vi "test_read-nmea-data2.vi"() -> ()   [LabVIEW 2019] (continued)
11,72,359,,2*70\n\t\n15:13:45.63\tF9P\t$GAGSV,2,2,08,12,40,103,,19,26,045,,25,09,249,,36,26,308,,2*7D\n\t\n15:13:45.65\tF9P\t$GBGSV,1,1,04,11,49,132,32,14,87,114,28,28,,,30,33,61,220,27,1*41\n\t\n15:13:45.67\tF9P\t$GBGSV,1,1,03,11,49,132,,14,87,114,27,33,61,220,,3*46\n\t\n15:13:45.69\tF9P\t$GNGLL,3723.57229,N,12656.98820,E,061347.00,A,A*73\n\t\n15:13:45.71\tF9P\t\t\n15:13:45.73\tF9P\t\t\n15:13:45.75\tF9P\t\t\n15:13:45.77\tF9P\t\t\n15:13:45.79\tF9P\t\t\n15:13:45.81\tF9P\t\t\n15:13:45.83\tF9P\t\t\n15:13:45.85\tF9P\t\t\n15:13:45.87\tF9P\t\t\n15:13:45.89\tF9P\t\t\n15:13:45.91\tF9P\t\t\n15:13:45.93\tF9P\t\t\n15:13:45.95\tF9P\t\t\n15:13:45.97\tF9P\t\t\n15:13:45.99\tF9P\t\t\n15:13:46.01\tF9P\t\t\n15:13:46.03\tF9P\t\t\n15:13:46.05\tF9P\t\t\n15:13:46.07\tF9P\t\t\n15:13:46.09\tF9P\t\t\n15:13:46.11\tF9P\t\t\n15:13:46.13\tF9P\t\t\n15:13:46.15\tF9P\t\t\n15:13:46.17\tF9P\t\t\n15:13:46.19\tF9P\t\t\n15:13:46.21\tF9P\t\t\n15:13:46.23\tF9P\t$GNRMC,061348.00,A,3723.57290,N,12656.98771,E,2.680,332.74,250720,,,A,V*07\n\t\n15:13:46.25\tF9P\t$GNVTG,332.74,T,,M,2.680,N,4.963,K,A*26\n\t\n15:13:46.27\tF9P\t$GNGGA,061348.00,3723.57290,N,12656.98771,E,1,12,0.78,48.0,M,18.5,M,,*7C\n\t\n15:13:46.29\tF9P\t$GNGSA,A,3,12,06,19,05,17,09,04,02,,,,,1.48,0.78,1.25,1*04\n\t\n15:13:46.31\tF9P\t$GNGSA,A,3,85,70,71,84,,,,,,,,,1.48,0.78,1.25,2*06\n\t\n15:13:46.33\tF9P\t$GNGSA,A,3,36,19,11,04,09,12,,,,,,,1.48,0.78,1.25,3*04\n\t\n15:13:46.35\tF9P\t$GNGSA,A,3,14,11,33,,,,,,,,,,1.48,0.78,1.25,4*05\n\t\n15:13:46.37\tF9P\t$GPGSV,3,1,09,02,55,320,32,04,17,043,25,05,38,248,28,06,64,050,31,1*66\n\t\n15:13:46.39\tF9P\t$GPGSV,3,2,09,09,44,073,30,12,23,276,41,17,32,154,36,19,51,157,34,1*6C\n\t\n15:13:46.41\tF9P\t$GPGSV,3,3,09,25,12,306,19,1*54\n\t\n15:13:46.43\tF9P\t$GPGSV,3,1,09,02,55,320,,04,17,043,14,05,38,248,18,06,64,050,24,6*65\n\t\n15:13:46.45\tF9P\t$GPGSV,3,2,09,09,44,073,24,12,23,276,22,17,32,154,22,19,51,157,,6*69\n\t\n15:13:46.47\tF9P\t$GPGSV,3,3,09,25,12,306,,6*5B\n\t\n15:13:46.49\tF9P\t$GLGSV,2,1,08,69,11,031,36,70,70,038,25,71,53,206,26,72,05,210,18,1*7D\n\t\n15:13:46.51\tF9P\t$GLGSV,2,2,08,77,01,325,,84,19,123,23,85,70,070,32,86,37,330,,1*76\n\t\n15:13:46.53\tF9P\t$GLGSV,2,1,08,69,11,031,25,70,70,038,,71,53,206,16,72,05,210,,3*70\n\t\n15:13:46.55\tF9P\t$GLGSV,2,2,08,77,01,325,,84,19,123,30,85,70,070,22,86,37,330,,3*77\n\t\n15:13:46.57\tF9P\t$GAGSV,2,1,08,02,08,297,10,04,66,116,32,09,32,193,24,11,72,359,26,7*77\n\t\n15:13:46.59\tF9P\t$GAGSV,2,2,08,12,40,103,25,19,26,045,16,25,09,249,19,36,26,308,17,7*76\n\t\n15:13:46.61\tF9P\t$GAGSV,2,1,08,02,08,297,,04,66,116,,09,32,193,,11,72,359,,2*70\n\t\n15:13:46.63\tF9P\t$GAGSV,2,2,08,12,40,103,,19,26,045,,25,09,249,,36,26,308,,2*7D\n\t\n15:13:46.65\tF9P\t$GBGSV,1,1,04,11,49,132,32,14,87,114,28,28,,,30,33,61,220,29,1*4F\n\t\n15:13:46.67\tF9P\t$GBGSV,1,1,03,11,49,132,31,14,87,114,27,33,61,220,,3*44\n\t\n15:13:46.69\tF9P\t$GNGLL,3723.57290,N,12656.98771,E,061348.00,A,A*75\n\t\n15:13:46.71\tF9P\t\t\n15:13:46.73\tF9P\t\t\n15:13:46.75\tF9P\t\t\n15:13:46.77\tF9P\t\t\n15:13:46.79\tF9P\t\t\n15:13:46.81\tF9P\t\t\n15:13:46.83\tF9P\t\t\n15:13:46.85\tF9P\t\t\n15:13:46.87\tF9P\t\t\n15:13:46.89\tF9P\t\t\n15:13:46.91\tF9P\t\t\n15:13:46.93\tF9P\t\t\n15:13:46.95\tF9P\t\t\n15:13:46.97\tF9P\t\t\n15:13:46.99\tF9P\t\t\n15:13:47.01\tF9P\t\t\n15:13:47.03\tF9P\t\t\n15:13:47.05\tF9P\t\t\n15:13:47.07\tF9P\t\t\n15:13:47.09\tF9P\t\t\n15:13:47.11\tF9P\t\t\n15:13:47.13\tF9P\t\t\n15:13:47.15\tF9P\t\t\n15:13:47.17\tF9P\t\t\n15:13:47.19\tF9P\t\t\n15:13:47.21\tF9P\t\t\n15:13:47.23\tF9P\t$GNRMC,061349.00,A,3723.57353,N,12656.98784,E,2.463,343.29,250720,,,A,V*03\n\t\n15:13:47.25\tF9P\t$GNVTG,343.29,T,,M,2.463,N,4.562,K,A*2A\n\t\n15:13:47.27\tF9P\t$GNGGA,061349.00,3723.57353,N,12656.98784,E,1,12,0.67,48.9,M,18.5,M,,*7E\n\t\n15:13:47.29\tF9P\t$GNGSA,A,3,12,06,19,05,17,09,04,02,,,,,1.24,0.67,1.04,1*03\n\t\n15:13:47.31\tF9P\t$GNGSA,A,3,85,70,71,84,,,,,,,,,1.24,0.67,1.04,2*01\n\t\n15:13:47.33\tF9P\t$GNGSA,A,3,36,19,11,04,09,12,,,,,,,1.24,0.67,1.04,3*03\n\t\n15:13:47.35\tF9P\t$GNGSA,A,3,14,11,33,,,,,,,,,,1.24,0.67,1.04,4*02\n\t\n15:13:47.37\tF9P\t$GPGSV,3,1,09,02,55,320,29,04,17,043,25,05,38,248,29,06,64,050,32,1*6E\n\t\n15:13:47.39\tF9P\t$GPGSV,3,2,09,09,44,073,25,12,23,276,41,17,32,154,28,19,51,157,37,1*64\n\t\n15:13:47.41\tF9P\t$GPGSV,3,3,09,25,12,306,18,1*55\n\t\n15:13:47.43\tF9P\t$GPGSV,3,1,09,02,55,320,,04,17,043,,05,38,248,18,06,64,050,25,6*61\n\t\n15:13:47.45\tF9P\t$GPGSV,3,2,09,09,44,073,25,12,23,276,24,17,32,154,22,19,51,157,,6*6E\n\t\n15:13:47.47\tF9P\t$GPGSV,3,3,09,25,12,306,,6*5B\n\t\n15:13:47.49\tF9P\t$GLGSV,2,1,08,69,11,031,31,70,70,038,24,71,53,206,26,72,05,210,19,1*7A\n\t\n15:13:47.51\tF9P\t$GLGSV,2,2,08,77,01,325,,84,19,123,24,85,70,070,31,86,37,330,,1*72\n\t\n15:13:47.53\tF9P\t$GLGSV,2,1,08,69,11,031,22,70,70,038,,71,53,206,15,72,05,210,,3*74\n\t\n15:13:47.55\tF9P\t$GLGSV,2,2,08,77,01,325,,84,19,123,22,85,70,070,22,86,37,330,,3*74\n\t\n15:13:47.57\tF9P\t$GAGSV,2,1,08,02,08,297,06,04,66,116,37,09,32,193,23,11,72,359,25,7*71\n\t\n15:13:47.59\tF9P\t$GAGSV,2,2,08,12,40,103,32,19,26,045,17,25,09,249,15,36,26,308,13,7*79\n\t\n15:13:47.61\tF9P\t$GAGSV,2,1,08,02,08,297,,04,66,116,,09,32,193,,11,72,359,,2*70\n\t\n15:13:47.63\tF9P\t$GAGSV,2,2,08,12,40,103,,19,26,045,,25,09,249,,36,26,308,,2*7D\n\t\n15:13:47.65\tF9P\t$GBGSV,1,1,04,11,49,132,27,14,87,114,28,28,,,30,33,61,220,38,1*4B\n\t\n15:13:47.67\tF9P\t$GBGSV,1,1,03,11,49,132,27,14,87,114,,33,61,220,,3*46\n\t\n15:13:47.69\tF9P\t$GNGLL,3723.57353,N,12656.98784,E,061349.00,A,A*70\n\t\n15:13:47.71\tF9P\t\t\n15:13:47.73\tF9P\t\t\n15:13:47.75\tF9P\t\t\n15:13:47.77\tF9P\t\t\n15:13:47.79\tF9P\t\t\n15:13:47.81\tF9P\t\t\n15:13:47.83\tF9P\t\t\n15:13:47.85\tF9P\t\t\n15:13:47.87\tF9P\t\t\n15:13:47.89\tF9P\t\t\n15:13:47.91\tF9P\t\t\n15:13:47.93\tF9P\t\t\n15:13:47.95\tF9P\t\t\n15:13:47.97\tF9P\t\t\n15:13:47.99\tF9P\t\t\n15:13:48.01\tF9P\t\t\n15:13:48.03\tF9P\t\t\n15:13:48.05\tF9P\t\t\n15:13:48.07\tF9P\t\t\n15:13:48.09\tF9P\t\t\n15:13:48.11\tF9P\t\t\n15:13:48.13\tF9P\t\t\n15:13:48.15\tF9P\t\t\n15:13:48.17\tF9P\t\t\n15:13:48.19\tF9P\t\t\n15:13:48.21\tF9P\t\t\n15:13:48.23\tF9P\t$GNRMC,061350.00,A,3723.57391,N,12656.98799,E,1.815,345.24,250720,,,A,V*0C\n\t\n15:13:48.25\tF9P\t$GNVTG,345.24,T,,M,1.815,N,3.361,K,A*2D\n\t\n15:13:48.27\tF9P\t$GNGGA,061350.00,3723.57391,N,12656.98799,E,1,12,0.75,49.6,M,18.5,M,,*79\n\t\n15:13:48.29\tF9P\t$GNGSA,A,3,12,06,19,05,17,09,04,02,,,,,1.37,0.75,1.15,1*02\n\t\n15:13:48.31\tF9P\t$GNGSA,A,3,85,70,71,84,,,,,,,,,1.37,0.75,1.15,2*00\n\t\n15:13:48.33\tF9P\t$GNGSA,A,3,36,19,11,04,09,12,,,,,,,1.37,0.75,1.15,3*02\n\t\n15:13:48.35\tF9P\t$GNGSA,A,3,14,11,33,,,,,,,,,,1.37,0.75,1.15,4*03\n\t\n15:13:48.37\tF9P\t$GPGSV,3,1,09,02,55,320,30,04,17,043,25,05,38,248,24,06,64,050,27,1*6F\n\t\n15:13:48.39\tF9P\t$GPGSV,3,2,09,09,44,073,32,12,23,276,34,17,32,154,36,19,51,157,32,1*6A\n\t\n15:13:48.41\tF9P\t$GPGSV,3,3,09,25,12,306,18,1*55\n\t\n15:13:48.43\tF9P\t$GPGSV,3,1,09,02,55,320,,04,17,043,,05,38,248,17,06,64,050,24,6*6F\n\t\n15:13:48.45\tF9P\t$GPGSV,3,2,09,09,44,073,25,12,23,276,24,17,32,154,21,19,51,157,,6*6D\n\t\n15:13:48.47\tF9P\t$GPGSV,3,3,09,25,12,306,,6*5B\n\t\n15:13:48.49\tF9P\t$GLGSV,2,1,08,69,11,031,29,70,70,038,25,71,53,206,27,72,05,210,19,1*73\n\t\n15:13:48.51\tF9P\t$GLGSV,2,2,08,77,01,325,,84,19,123,25,85,70,070,31,86,37,330,,1*73\n\t\n15:13:48.53\tF9P\t$GLGSV,2,1,08,69,11,031,21,70,70,038,,71,53,206,14,72,05,210,,3*76\n\t\n15:13:48.55\tF9P\t$GLGSV,2,2,08,77,01,325,,84,19,123,23,85,70,070,21,86,37,330,,3*76\n\t\n15:13:48.57\tF9P\t$GAGSV,2,1,08,02,08,297,10,04,66,116,36,09,32,193,22,11,72,359,25,7*76\n\t\n15:13:48.59\tF9P\t$GAGSV,2,2,08,12,40,103,30,19,26,045,16,25,09,249,14,36,26,308,12,7*7A\n\t\n15:13:48.61\tF9P\t$GAGSV,2,1,08,02,08,297,,04,66,116,,09,32,193,,11,72,359,,2*70\n\t\n15:13:48.63\tF9P\t$GAGSV,2,2,08,12,40,103,,19,26,045,,25,09,249,,36,26,308,,2*7D\n\t\n15:13:48.65\tF9P\t$GBGSV,1,1,04,11,49,132,32,14,87,114,28,28,,,35,33,61,220,33,1*41\n\t\n15:13:48.67\tF9P\t$GBGSV,1,1,03,11,49,132,26,14,87,114,,33,61,220,,3*47\n\t\n15:13:48.69\tF9P\t$GNGLL,3723.57391,N,12656.98799,E,061350.00,A,A*7A\n\t\n15:13:48.71\tF9P\t\t\n15:13:48.73\tF9P\t\t\n15:13:48.75\tF9P\t\t\n15:13:48.77\tF9P\t\t\n15:13:48.79\tF9P\t\t\n15:13:48.81\tF9P\t\t\n15:13:48.83\tF9P\t\t\n15:13:48.85\tF9P\t\t\n15:13:48.87\tF9P\t\t\n15:13:48.89\tF9P\t\t\n15:13:48.91\tF9P\t\t\n15:13:48.93\tF9P\t\t\n15:13:48.95\tF9P\t\t\n15:13:48.97\tF9P\t\t\n15:13:48.99\tF9P\t\t\n15:13:49.01\tF9P\t\t\n15:13:49.03\tF9P\t\t\n15:13:49.05\tF9P\t\t\n15:13:49.07\tF9P\t\t\n15:13:49.09\tF9P\t\t\n15:13:49.11\tF9P\t\t\n15:13:49.13\tF9P\t\t\n15:13:49.15\tF9P\t\t\n15:13:49.17\tF9P\t\t\n15:13:49.19\tF9P\t\t\n15:13:49.21\tF9P\t\t\n15:13:49.23\tF9P\t$GNRMC,061351.00,A,3723.57445,N,12656.98793,E,1.823,343.63,250720,,,A,V*09\n\t\n15:13:49.25\tF9P\t$GNVTG,343.63,T,,M,1.823,N,3.376,K,A*2B\n\t\n15:13:49.27\tF9P\t$GNGGA,061351.00,3723.57445,N,12656.98793,E,1,12,0.70,49.5,M,18.5,M,,*7A\n\t\n15:13:49.29\tF9P\t$GNGSA,A,3,12,06,19,05,17,09,04,02,,,,,1.27,0.70,1.06,1*04\n\t\n15:13:49.31\tF9P\t$GNGSA,A,3,85,70,71,84,,,,,,,,,1.27,0.70,1.06,2*06\n\t\n15:13:49.33\tF9P\t$GNGSA,A,3,36,19,11,04,09,12,,,,,,,1.27,0.70,1.06,3*04\n\t\n15:13:49.35\tF9P\t$GNGSA,A,3,14,11,33,,,,,,,,,,1.27,0.70,1.06,4*05\n\t\n15:13:49.37\tF9P\t$GPGSV,3,1,09,02,55,320,29,04,17,043,25,05,38,248,34,06,64,050,28,1*69\n\t\n15:13:49.39\tF9P\t$GPGSV,3,2,09,09,44,073,28,12,23,276,33,17,32,154,29,19,51,157,36,1*6C\n\t\n15:13:49.41\tF9P\t$GPGSV,3,3,09,25,12,306,21,1*5F\n\t\n15:13:49.43\tF9P\t$GPGSV,3,1,09,02,55,320,,04,17,043,,05,38,248,17,06,64,050,22,6*69\n\t\n15:13:49.45\tF9P\t$GPGSV,3,2,09,09,44,073,24,12,23,276,22,17,32,154,20,19,51,157,,6*6B\n\t\n15:13:49.47\tF9P\t$GPGSV,3,3,09,25,12,306,,6*5B\n\t\n15:13:49.49\tF9P\t$GLGSV,2,1,08,69,11,031,30,70,70,038,24,71,53,206,27,72,05,210,18,1*7B\n\t\n15:13:49.51\tF9P\t$GLGSV,2,2,08,77,01,325,,84,19,123,24,85,70,070,27,86,37,330,,1*75\n\t\n15:13:49.53\tF9P\t$GLGSV,2,1,08,69,11,031,21,70,70,038,,71,53,206,14,72,05,210,,3*76\n\t\n15:13:49.55\tF9P\t$GLGSV,2,2,08,77,01,325,,84,19,123,24,85,70,070,21,86,37,330,,3*71\n\t\n15:13:49.57\tF9P\t$GAGSV,2,1,08,02,08,296,09,04,66,116,30,09,32,193,22,11,72,359,24,7*78\n\t\n15:13:49.59\tF9P\t$GAGSV,2,2,08,12,40,103,34,19,26,045,16,25,09,249,13,36,26,308,12,7*79\n\t\n15:13:49.61\tF9P\t$GAGSV,2,1,08,02,08,296,,04,66,116,,09,32,193,,11,72,359,,2*71\n\t\n15:13:49.63\tF9P\t$GAGSV,2,2,08,12,40,103,,19,26,045,,25,09,249,,36,26,308,,2*7D\n\t\n15:13:49.65\tF9P\t$GBGSV,1,1,04,11,49,132,39,14,87,114,28,28,,,27,33,61,220,39,1*43\n\t\n15:13:49.67\tF9P\t$GBGSV,1,1,03,11,49,132,,14,87,114,,33,61,220,,3*43\n\t\n15:13:49.69\tF9P\t$GNGLL,3723.57445,N,12656.98793,E,061351.00,A,A*7F\n\t\n15:13:49.71\tF9P\t\t\n15:13:49.73\tF9P\t\t\n15:13:49.75\tF9P\t\t\n15:13:49.77\tF9P\t\t\n15:13:49.79\tF9P\t\t\n15:13:49.81\tF9P\t\t\n15:13:49.83\tF9P\t\t\n15:13:49.85\tF9P\t\t\n15:13:49.87\tF9P\t\t\n15:13:49.89\tF9P\t\t\n15:13:49.91\tF9P\t\t\n15:13:49.93\tF9P\t\t\n15:13:49.95\tF9P\t\t\n15:13:49.97\tF9P\t\t\n15:13:49.99\tF9P\t\t\n15:13:50.01\tF9P\t\t\n15:13:50.03\tF9P\t\t\n15:13:50.05\tF9P\t\t\n15:13:50.07\tF9P\t\t\n15:13:50.09\tF9P\t\t\n15:13:50.11\tF9P\t\t\n15:13:50.13\tF9P\t\t\n15:13:50.15\tF9P\t\t\n15:13:50.17\tF9P\t\t\n15:13:50.19\tF9P\t\t\n15:13:50.21\tF9P\t\t\n15:13:50.23\tF9P\t$GNRMC,061352.00,A,3723.57495,N,12656.98774,E,1.787,343.52,250720,,,A,V*0D\n\t\n15:13:50.25\tF9P\t$GNVTG,343.52,T,,M,1.787,N,3.310,K,A*28\n\t\n15:13:50.27\tF9P\t$GNGGA,061352.00,3723.57495,N,12656.98774,E,1,12,0.81,49.2,M,18.5,M,,*74\n\t\n15:13:50.29\tF9P\t$GNGSA,A,3,12,06,19,05,17,09,04,02,,,,,1.45,0.81,1.20,1*0A\n\t\n15:13:50.31\tF9P\t$GNGSA,A,3,85,70,71,84,,,,,,,,,1.45,0.81,1.20,2*08\n\t\n15:13:50.33\tF9P\t$GNGSA,A,3,36,19,11,04,09,12,,,,,,,1.45,0.81,1.20,3*0A\n\t\n15:13:50.35\tF9P\t$GNGSA,A,3,14,11,33,,,,,,,,,,1.45,0.81,1.20,4*0B\n\t\n15:13:50.37\tF9P\t$GPGSV,3,1,09,02,55,320,30,04,17,043,24,05,38,248,,06,64,050,29,1*66\n\t\n15:13:50.39\tF9P\t$GPGSV,3,2,09,09,44,073,29,12,23,276,32,17,32,154,33,19,51,157,41,1*67\n\t\n15:13:50.41\tF9P\t$GPGSV,3,3,09,25,12,306,24,1*5A\n\t\n15:13:50.43\tF9P\t$GPGSV,3,1,09,02,55,320,,04,17,043,,05,38,248,15,06,64,050,23,6*6A\n\t\n15:13:50.45\tF9P\t$GPGSV,3,2,09,09,44,073,22,12,23,276,21,17,32,154,19,19,51,157,,6*64\n\t\n15:13:50.47\tF9P\t$GPGSV,3,3,09,25,12,306,,6*5B\n\t\n15:13:50.49\tF9P\t$GLGSV,2,1,08,69,11,031,31,70,70,038,24,71,53,206,32,72,05,210,18,1*7E\n\t\n15:13:50.51\tF9P\t$GLGSV,2,2,08,77,01,325,,84,19,123,25,85,70,070,32,86,37,330,,1*70\n\t\n15:13:50.53\tF9P\t$GLGSV,2,1,08,69,11,031,23,70,70,038,,71,53,206,16,72,05,210,,3*76\n\t\n15:13:50.55\tF9P\t$GLGSV,2,2,08,77,01,325,,84,19,123,26,85,70,070,19,86,37,330,,3*78\n\t\n15:13:50.57\tF9P\t$GAGSV,2,1,08,02,08,296,09,04,66,116,28,09,32,193,20,11,72,359,26,7*71\n\t\n15:13:50.59\tF9P\t$GAGSV,2,2,08,12,40,103,29,19,26,045,15,25,09,249,13,36,26,308,10,7*74\n\t\n15:13:50.61\tF9P\t$GAGSV,2,1,08,02,08,296,,04,66,116,,09,32,193,,11,72,359,,2*71\n\t\n15:13:50.63\tF9P\t$GAGSV,2,2,08,12,40,103,,19,26,045,,25,09,249,,36,26,308,,2*7D\n\t\n15:13:50.65\tF9P\t$GBGSV,1,1,04,11,49,132,37,14,87,114,29,28,,,32,33,61,220,29,1*49\n\t\n15:13:50.67\tF9P\t$GBGSV,1,1,03,11,49,132,29,14,87,114,,33,61,220,,3*48\n\t\n15:13:50.69\tF9P\t$GNGLL,3723.57495,N,12656.98774,E,061352.00,A,A*78\n\t\n15:13:50.71\tF9P\t\t\n15:13:50.73\tF9P\t\t\n15:13:50.75\tF9P\t\t\n15:13:50.77\tF9P\t\t\n15:13:50.79\tF9P\t\t\n15:13:50.81\tF9P\t\t\n15:13:50.83\tF9P\t\t\n15:13:50.85\tF9P\t\t\n15:13:50.87\tF9P\t\t\n15:13:50.89\tF9P\t\t\n15:13:50.91\tF9P\t\t\n15:13:50.93\tF9P\t\t\n15:13:50.95\tF9P\t\t\n15:13:50.97\tF9P\t\t\n15:13:50.99\tF9P\t\t\n15:13:51.01\tF9P\t\t\n15:13:51.03\tF9P\t\t\n15:13:51.05\tF9P\t\t\n15:13:51.07\tF9P\t\t\n15:13:51.09\tF9P\t\t\n15:13:51.11\tF9P\t\t\n15:13:51.13\tF9P\t\t\n15:13:51.15\tF9P\t\t\n15:13:51.17\tF9P\t\t\n15:13:51.19\tF9P\t\t\n15:13:51.21\tF9P\t\t\n15:13:51.23\tF9P\t$GNRMC,061353.00,A,3723.57578,N,12656.98744,E,2.592,340.93,250720,,,A,V*06\n\t\n15:13:51.25\tF9P\t$GNVTG,340.93,T,,M,2.592,N,4.801,K,A*2F\n\t\n15:13:51.27\tF9P\t$GNGGA,061353.00,3723.57578,N,12656.98744,E,1,12,0.81,49.0,M,18.5,M,,*76\n\t\n15:13:51.29\tF9P\t$GNGSA,A,3,12,06,19,05,17,09,04,02,,,,,1.45,0.81,1.20,1*0A\n\t\n15:13:51.31\tF9P\t$GNGSA,A,3,85,70,71,84,,,,,,,,,1.45,0.81,1.20,2*08\n\t\n15:13:51.33\tF9P\t$GNGSA,A,3,36,19,11,04,09,12,,,,,,,1.45,0.81,1.20,3*0A\n\t\n15:13:51.35\tF9P\t$GNGSA,A,3,14,11,33,,,,,,,,,,1.45,0.81,1.20,4*0B\n\t\n15:13:51.37\tF9P\t$GPGSV,3,1,09,02,55,320,28,04,17,043,23,05,38,248,25,06,64,050,28,1*6E\n\t\n15:13:51.39\tF9P\t$GPGSV,3,2,09,09,44,073,30,12,23,276,25,17,32,154,30,19,51,157,42,1*69\n\t\n15:13:51.41\tF9P\t$GPGSV,3,3,09,25,12,306,25,1*5B\n\t\n15:13:51.43\tF9P\t$GPGSV,3,1,09,02,55,320,,04,17,043,,05,38,248,16,06,64,050,29,6*63\n\t\n15:13:51.45\tF9P\t$GPGSV,3,2,09,09,44,073,22,12,23,276,18,17,32,154,19,19,51,157,,6*6E\n\t\n15:13:51.47\tF9P\t$GPGSV,3,3,09,25,12,306,,6*5B\n\t\n15:13:51.49\tF9P\t$GLGSV,2,1,08,69,11,031,31,70,70,038,24,71,53,206,32,72,05,210,16,1*70\n\t\n15:13:51.51\tF9P\t$GLGSV,2,2,08,77,01,325,,84,19,123,30,85,70,070,26,86,37,330,,1*71\n\t\n15:13:51.53\tF9P\t$GLGSV,2,1,08,69,11,031,24,70,70,038,,71,53,206,19,72,05,210,,3*7E\n\t\n15:13:51.55\tF9P\t$GLGSV,2,2,08,77,01,325,,84,19,123,31,85,70,070,19,86,37,330,,3*7E\n\t\n15:13:51.57\tF9P\t$GAGSV,2,1,08,02,08,296,06,04,67,115,28,09,32,193,21,11,72,359,27,7*7C\n\t\n15:13:51.59\tF9P\t$GAGSV,2,2,08,12,40,103,28,19,26,045,16,25,09,249,13,36,26,308,13,7*75\n\t\n15:13:51.61\tF9P\t$GAGSV,2,1,08,02,08,296,,04,67,115,,09,32,193,,11,72,359,,2*73\n\t\n15:13:51.63\tF9P\t$GAGSV,2,2,08,12,40,103,,19,26,045,,25,09,249,,36,26,308,,2*7D\n\t\n15:13:51.65\tF9P\t$GBGSV,1,1,04,11,49,132,41,14,87,114,27,28,,,32,33,61,220,39,1*47\n\t\n15:13:51.67\tF9P\t$GBGSV,1,1,03,11,49,132,33,14,87,114,,33,61,220,,3*43\n\t\n15:13:51.69\tF9P\t$GNGLL,3723.57578,N,12656.98744,E,061353.00,A,A*78\n\t\n15:13:51.71\tF9P\t\t\n15:13:51.73\tF9P\t\t\n15:13:51.75\tF9P\t\t\n15:13:51.77\tF9P\t\t\n15:13:51.79\tF9P\t\t\n15:13:51.81\tF9P\t\t\n15:13:51.83\tF9P\t\t\n15:13:51.85\tF9P\t\t\n15:13:51.87\tF9P\t\t\n15:13:51.89\tF9P\t\t\n15:13:51.91\tF9P\t\t\n15:13:51.93\tF9P\t\t\n15:13:51.95\tF9P\t\t\n15:13:51.97\tF9P\t\t\n15:13:51.99\tF9P\t\t\n15:13:52.01\tF9P\t\t\n15:13:52.03\tF9P\t\t\n15:13:52.05\tF9P\t\t\n15:13:52.07\tF9P\t\t\n15:13:52.09\tF9P\t\t\n15:13:52.11\tF9P\t\t\n15:13:52.13\tF9P\t\t\n15:13:52.15\tF9P\t\t\n15:13:52.17\tF9P\t\t\n15:13:52.19\tF9P\t\t\n15:13:52.21\tF9P\t\t\n15:13:52.23\tF9P\t$GNRMC,061354.00,A,3723.57605,N,12656.98738,E,1.756,335.43,250720,,,A,V*05\n\t\n15:13:52.25\tF9P\t$GNVTG,335.43,T,,M,1.756,N,3.252,K,A*22\n\t\n15:13:52.27\tF9P\t$GNGGA,061354.00,3723.57605,N,12656.98738,E,1,12,0.70,50.3,M,18.5,M,,*76\n\t\n15:13:52.29\tF9P\t$GNGSA,A,3,12,06,19,05,17,09,04,02,,,,,1.27,0.70,1.06,1*04\n\t\n15:13:52.31\tF9P\t$GNGSA,A,3,85,70,71,84,,,,,,,,,1.27,0.70,1.06,2*06\n\t\n15:13:52.33\tF9P\t$GNGSA,A,3,36,19,11,04,09,12,,,,,,,1.27,0.70,1.06,3*04\n\t\n15:13:52.35\tF9P\t$GNGSA,A,3,14,11,33,,,,,,,,,,1.27,0.70,1.06,4*05\n\t\n15:13:52.37\tF9P\t$GPGSV,3,1,09,02,55,320,27,04,17,043,22,05,38,248,36,06,64,050,29,1*63\n\t\n15:13:52.39\tF9P\t$GPGSV,3,2,09,09,44,073,33,12,23,276,27,17,32,154,36,19,51,157,40,1*6C\n\t\n15:13:52.41\tF9P\t$GPGSV,3,3,09,25,12,306,25,1*5B\n\t\n15:13:52.43\tF9P\t$GPGSV,3,1,09,02,55,320,,04,17,043,,05,38,248,15,06,64,050,23,6*6A\n\t\n15:13:52.45\tF9P\t$GPGSV,3,2,09,09,44,073,24,12,23,276,17,17,32,154,20,19,51,157,,6*6D\n\t\n15:13:52.47\tF9P\t$GPGSV,3,3,09,25,12,306,,6*5B\n\t\n15:13:52.49\tF9P\t$GLGSV,2,1,08,69,11,031,32,70,70,038,25,71,53,206,31,72,05,210,16,1*71\n\t\n15:13:52.51\tF9P\t$GLGSV,2,2,08,77,01,325,,84,19,123,22,85,70,070,32,86,37,330,,1*77\n\t\n15:13:52.53\tF9P\t$GLGSV,2,1,08,69,11,031,23,70,70,038,,71,53,206,22,72,05,210,,3*71\n\t\n15:13:52.55\tF9P\t$GLGSV,2,2,08,77,01,325,,84,19,123,30,85,70,070,22,86,37,330,,3*77\n\t\n15:13:52.57\tF9P\t$GAGSV,2,1,08,02,08,296,10,04,67,115,27,09,32,193,20,11,72,359,27,7*75\n\t\n15:13:52.59\tF9P\t$GAGSV,2,2,08,12,40,103,33,19,26,045,18,25,09,249,12,36,26,308,12,7*71\n\t\n15:13:52.61\tF9P\t$GAGSV,2,1,08,02,08,296,,04,67,115,,09,32,193,,11,72,359,,2*73\n\t\n15:13:52.63\tF9P\t$GAGSV,2,2,08,12,40,103,,19,26,045,,25,09,249,,36,26,308,,2*7D\n\t\n15:13:52.65\tF9P\t$GBGSV,1,1,04,11,49,132,33,14,87,114,32,28,,,27,33,61,220,32,1*49\n\t\n15:13:52.67\tF9P\t$GBGSV,1,1,03,11,49,132,33,14,87,114,,33,61,220,,3*43\n\t\n15:13:52.69\tF9P\t$GNGLL,3723.57605,N,12656.98738,E,061354.00,A,A*7D\n\t\n15:13:52.71\tF9P\t\t\n15:13:52.73\tF9P\t\t\n15:13:52.75\tF9P\t\t\n15:13:52.77\tF9P\t\t\n15:13:52.79\tF9P\t\t\n15:13:52.81\tF9P\t\t\n15:13:52.83\tF9P\t\t\n15:13:52.85\tF9P\t\t\n15:13:52.87\tF9P\t\t\n15:13:52.89\tF9P\t\t\n15:13:52.91\tF9P\t\t\n15:13:52.93\tF9P\t\t\n15:13:52.95\tF9P\t\t\n15:13:52.97\tF9P\t\t\n15:13:52.99\tF9P\t\t\n15:13:53.01\tF9P\t\t\n15:13:53.03\tF9P\t\t\n15:13:53.05\tF9P\t\t\n15:13:53.07\tF9P\t\t\n15:13:53.09\tF9P\t\t\n15:13:53.11\tF9P\t\t\n15:13:53.13\tF9P\t\t\n15:13:53.15\tF9P\t\t\n15:13:53.17\tF9P\t\t\n15:13:53.19\tF9P\t\t\n15:13:53.21\tF9P\t\t\n15:13:53.23\tF9P\t$GNRMC,061355.00,A,3723.57673,N,12656.98677,E,2.481,323.44,250720,,,A,V*05\n\t\n15:13:53.25\tF9P\t$GNVTG,323.44,T,,M,2.481,N,4.595,K,A*23\n\t\n15:13:53.27\tF9P\t$GNGGA,061355.00,3723.57673,N,12656.98677,E,1,12,0.74,49.6,M,18.5,M,,*75\n\t\n15:13:53.29\tF9P\t$GNGSA,A,3,12,06,19,05,17,09,04,02,,,,,1.37,0.74,1.15,1*03\n\t\n15:13:53.31\tF9P\t$GNGSA,A,3,85,70,71,84,,,,,,,,,1.37,0.74,1.15,2*01\n\t\n15:13:53.33\tF9P\t$GNGSA,A,3,36,19,11,04,09,12,,,,,,,1.37,0.74,1.15,3*03\n\t\n15:13:53.35\tF9P\t$GNGSA,A,3,14,11,33,,,,,,,,,,1.37,0.74,1.15,4*02\n\t\n15:13:53.37\tF9P\t$GPGSV,3,1,09,02,55,320,31,04,17,043,23,05,38,248,39,06,64,050,29,1*6A\n\t\n15:13:53.39\tF9P\t$GPGSV,3,2,09,09,44,073,40,12,23,276,27,17,32,154,33,19,51,157,39,1*63\n\t\n15:13:53.41\tF9P\t$GPGSV,3,3,09,25,12,306,25,1*5B\n\t\n15:13:53.43\tF9P\t$GPGSV,3,1,09,02,55,320,,04,17,043,,05,38,248,18,06,64,050,24,6*60\n\t\n15:13:53.45\tF9P\t$GPGSV,3,2,09,09,44,073,23,12,23,276,15,17,32,154,19,19,51,157,,6*62\n\t\n15:13:53.47\tF9P\t$GPGSV,3,3,09,25,12,306,,6*5B\n\t
